vi "New Received Waveform.vi"(6 "Wfm Index":i32, 8 "error in (no error)":errorcluster, 9 "Associated Logs":T1[](array[typedef]), 10 "Buffer data?":bool, 11 "Wfm Buffer Ref":refnum<data-value>) -> (0 "error out":errorcluster, 3 "Waveform Receive out":refnum<class "Waveform Receive.lvclass">)   [LabVIEW 2015, in "Waveform Receive.lvclass"]
uses:
  Waveform Receive.lvclass
  Buffer/Waveform Buffer/Waveform Buffer.lvclass
  Associated Log.ctl
  Waveform Receive.lvclass/Waveform Receive.ctl
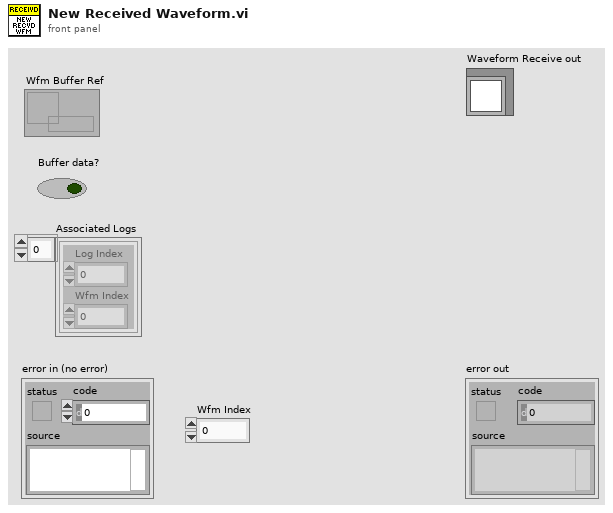
[diagram p1: front panel]
types:
  T1 = typedef "Waveform Receive.lvclass/Associated Log.ctl" = cluster{"Log Index":i32, "Wfm Index":i32}
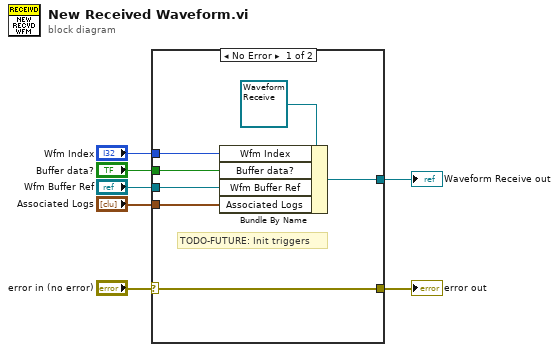
[diagram p0: block diagram]
diagram:
  n1 = case shown="No Error" "error in (no error)" {
    selector: "error in (no error)" -> [w14 w15]
    tunnel: [w14 w15] -> w6
    tunnel: [w12 _] -> w5
    tunnel: "Associated Logs" -> [w11 _]
    tunnel: "Wfm Buffer Ref" -> [w10 _]
    tunnel: "Buffer data?" -> [w9 _]
    tunnel: "Wfm Index" -> [w8 _]
    frame No Error {
      # "TODO-FUTURE: Init triggers"
      n2 = Bundle By Name(cluster=refnum<class "Waveform Receive.lvclass"> refnum ("Waveform Receive in"), "Wfm Index"=w8, "Buffer data?"=w9, "Wfm Buffer Ref"=w10, "Associated Logs"=w11) -> (w12:refnum<class "Waveform Receive.lvclass">)
    }
    frame Error {
    }
  }
  "error out" <- w6
  "Waveform Receive out" <- w5
